vi "TCV1.vi"() -> ()   [LabVIEW 2024]
uses:
  <vilib>/vision/driver/NI_Vision_Acquisition_Software.lvlib
  dependencies_dll_release/TCV_Lib.dll
  <resource>/objmgr/imaqdx.rc
panel:
  in  "CPU:0/Gpu:1":i32=1
  in  "Class name path":path=path "D:/labviewTestTCVdll/TransformCV-LabVIEW/Test/model/candyClasses.txt"
  out "Device Num":u64
  out "success_model_loading":u64
  in  "Model Path":path=path "D:/labviewTestTCVdll/TransformCV-LabVIEW/Test/model/candy11s_1_3_736_1280_gpu.torchscript"
  in  "model_h":i32=736
  in  "iou":dbl=0.65
  in  "conf":dbl=0.6100000000000001 min=0.01 max=1.0 step=0.05
  in  "model_w":i32=1280
  out "height":u32
  out "width":u32
  out "video Mode names":string[](array[string])
  in  "Resolution Selection":u16(ring)=10 items=["640x480 MJPG 30.00fps", "1280x720 MJPG 30.00fps", "1920x1080 MJPG 30.00fps", "1920x1088 MJPG 30.00fps"]
  in  "Camera Selection":string(combo)="cam5"
  in  "confirm camera":bool
  out "Camera Index list":string[](array[string])
  out "Camera":T1(plugin-control)
  in  "stop":bool
  out "return type":i32
  out "no_of_detections":i32
  out "arry_cluster":T2(array[cluster])
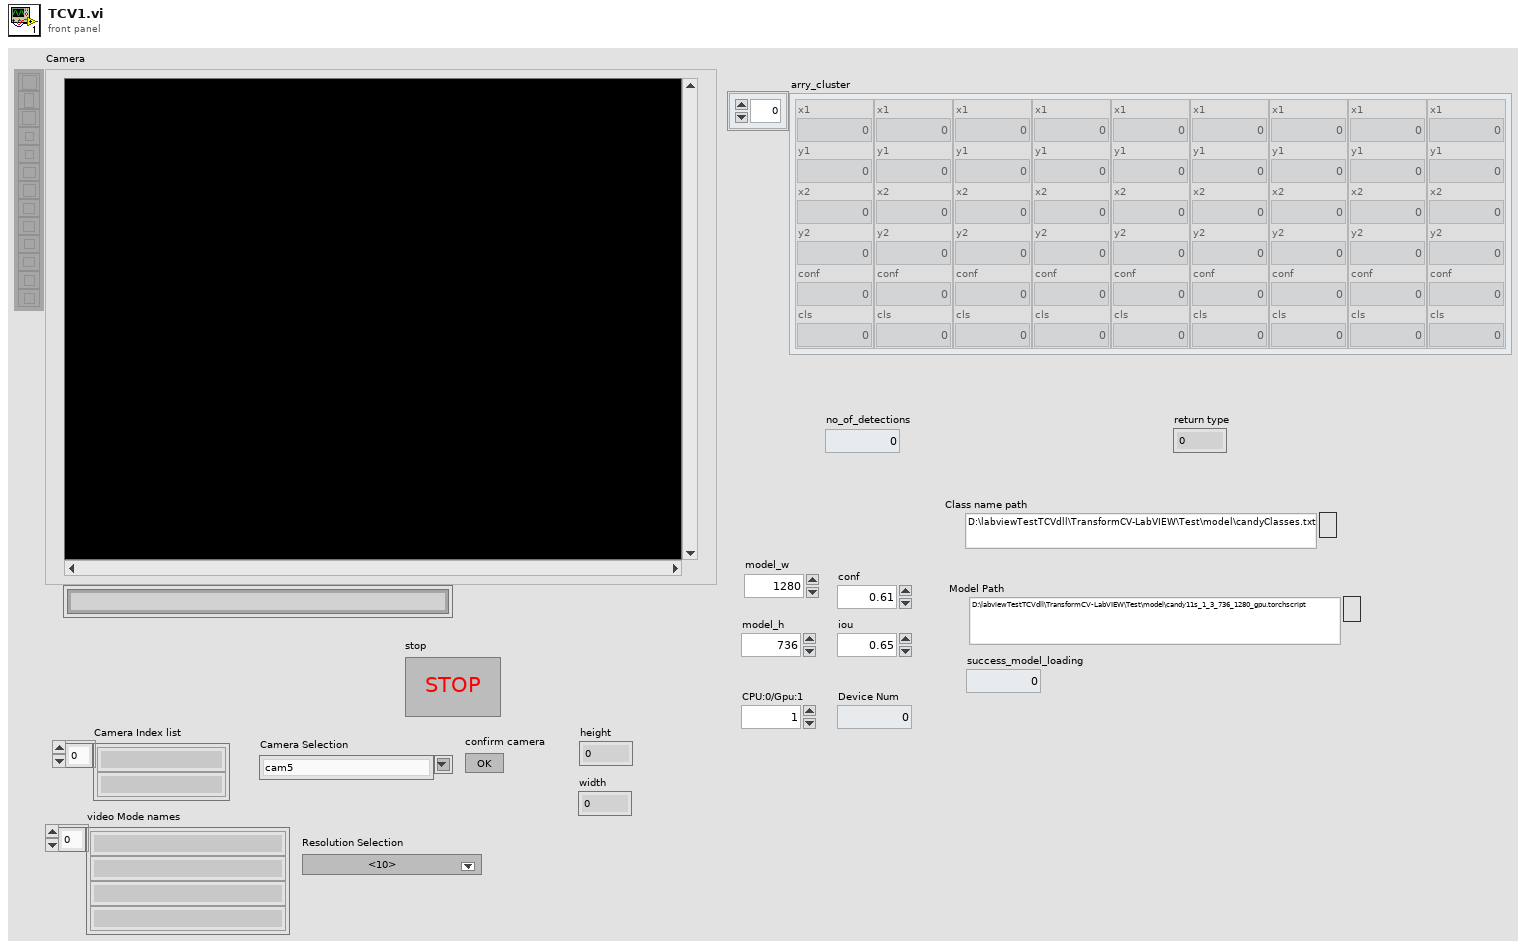
[diagram p1: front panel]
types:
  T1 = typedef "IMAQ Image.ctl" = refnum<image>
  T2 = cluster{"x1":sgl, "y1":sgl, "x2":sgl, "y2":sgl, "conf":sgl, "cls":i32}[]
  T3 = cluster{"Type":u32, "Version":u32, "Flags":u32, "SerialNumberHigh":u32, "SerialNumberLow":u32, "BusType":u32, "InterfaceName":string, "VendorName":string, "ModelName":string, "CameraFileName":string, "CameraAttributeURL":string}[]
  T4 = typedef "IMAQdx.ctl" = refnum<k21>
  T5 = cluster{"Video Mode":u32, "Video Mode Name":string}[]
  T6 = cluster{"x1":sgl, "y1":sgl, "x2":sgl, "y2":sgl, "conf":sgl, "cls":i32}
  T7 = enum32{"Map Pixel Pointer", "Unmap Pixel Pointer", "Get Pixels Infos"}
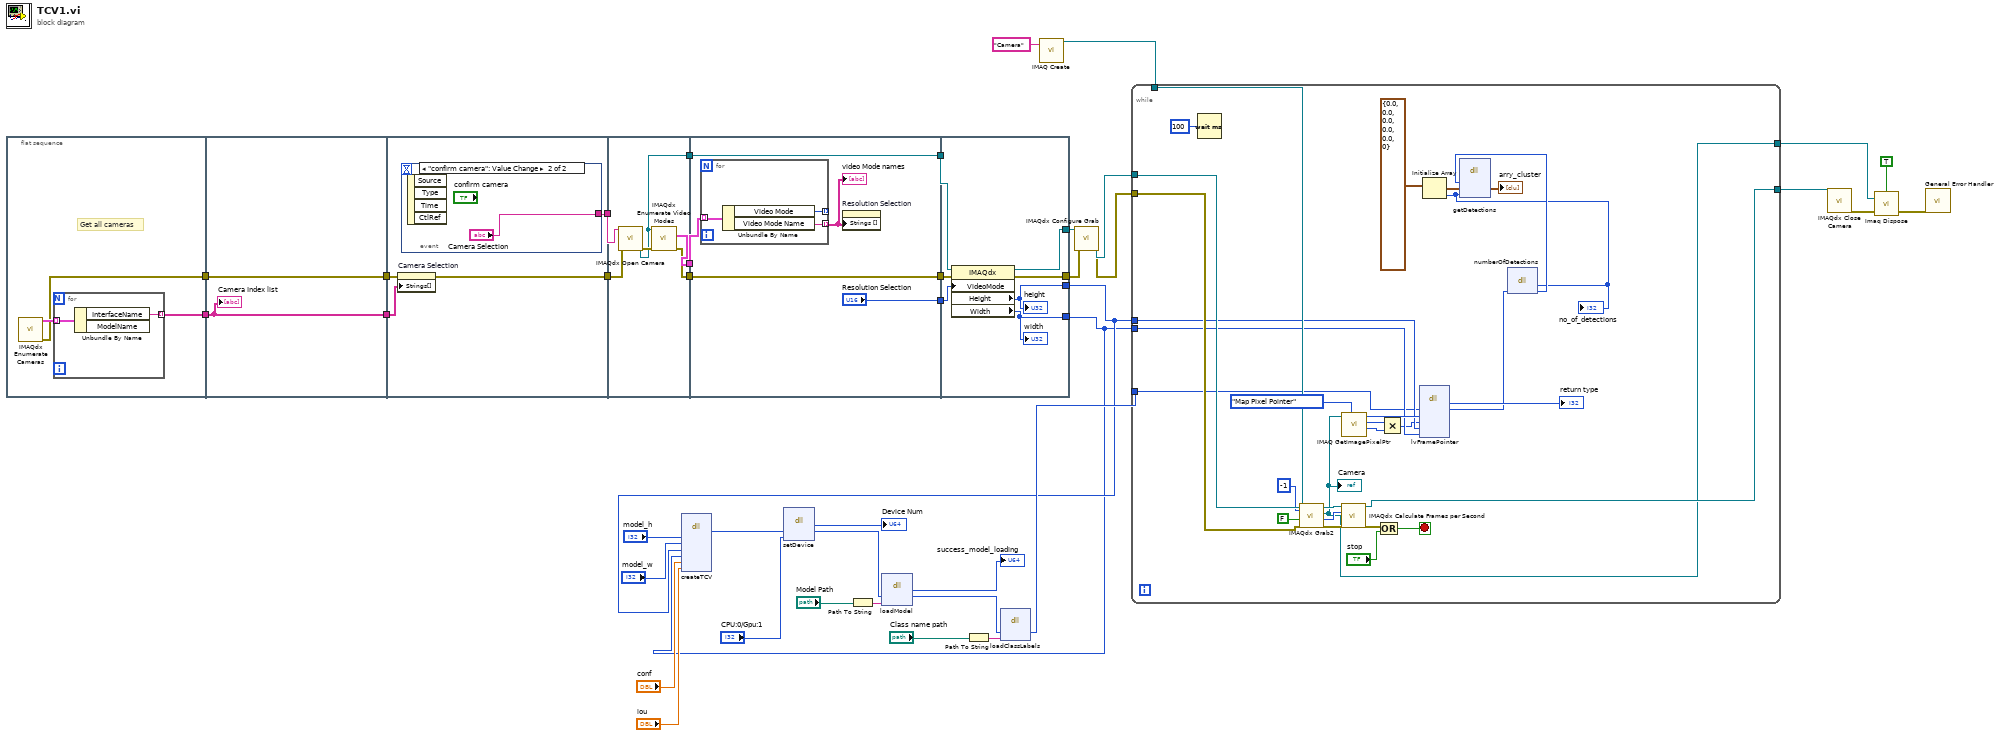
[diagram p0: block diagram]
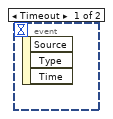
[diagram p2: hidden frame]
diagram:
  n1 = flat-sequence {
    tunnel: [w43] -> w40
    tunnel: [w41] -> w39
    tunnel: w40 -> [w47]
    tunnel: [w47] -> w38
    tunnel: [w46] -> w37
    tunnel: w39 -> [w46]
    tunnel: w38 -> [w51]
    tunnel: w37 -> [w50]
    tunnel: [w48] -> w36
    tunnel: [w49] -> w35
    tunnel: w36 -> [w58]
    tunnel: w35 -> [w57]
    tunnel: [w55] -> w34
    tunnel: [w54] -> w33
    tunnel: [w53] -> w32
    tunnel: w34 -> [w63]
    tunnel: [w61] -> w31
    tunnel: w33 -> [w61]
    tunnel: ["Resolution Selection"] -> w30
    tunnel: [w59] -> w29
    tunnel: w32 -> [w59]
    tunnel: w31 -> [w73]
    tunnel: w30 -> [w72]
    tunnel: w29 -> [w71]
    tunnel: [w70] -> w1
    tunnel: [w69] -> w2
    tunnel: [w68] -> w19
    tunnel: [w67] -> w18
    frame #0 {
      # "Get all cameras"
      n2 = call <vilib>:"IMAQdx Enumerate Cameras.vi"() -> ("error out"=w41:errorcluster, "Camera Information Array"=w42:T3)  [unwired: 10 in]
      n3 = for {
        tunnel: w42 -> [w45] mode=indexing
        tunnel: [w44] -> w43 mode=indexing
        n4 = Unbundle By Name(w45) -> ("InterfaceName"=w44:string)  [unwired: 1 out]
      }
    }
    frame #1 {
      "Camera Index list" <- w47
    }
    frame #2 {
      n5 = property on="Camera Selection" class="CmbBox"(error in=w50, "Strings[]"=w51) -> (error out=w49:errorcluster)  [unwired: 1 in, 1 out]
      n6 = event shown="[1] \"confirm camera\": Value Change" {
        selector: _ -> [_ _]
        dyn-events: _ -> [_ _]
        timeout: _ -> [_ _]
        tunnel: [_ "Camera Selection"] -> w48
        event Timeout {
          n7 = event-data() -> ()  [unwired: 1 in, 3 out]
        }
        event "confirm camera": Value Change {
          n8 = event-data() -> ()  [unwired: 1 in, 4 out]
        }
      }
    }
    frame #3 {
      n9 = call <vilib>:"IMAQdx Open Camera.vi"("error in"=w57, "Session In"=w58) -> ("error out"=w56:errorcluster, "Session Out"=w54:T4)  [unwired: 8 in]
      n10 = call <vilib>:"IMAQdx Enumerate Video Modes.vi"("error in"=w56, "Session In"=w54) -> ("error out"=w53:errorcluster, "Video Modes"=w55:T5)  [unwired: 6 in, 2 out]
    }
    frame #4 {
      n11 = for {
        tunnel: w63 -> [w66] mode=indexing
        tunnel: [w65] -> _ mode=indexing
        tunnel: [w64] -> w62 mode=indexing
        n12 = Unbundle By Name(w66) -> ("Video Mode"=w65:u32, "Video Mode Name"=w64:string)
      }
      "video Mode names" <- w62
      n13 = property on="Resolution Selection" class="Ring (strict)"("Strings []"=w62) -> ()  [unwired: 2 in, 2 out]
    }
    frame #5 {
      n14 = property class="IMAQdx"(reference=w73, error in=w71, "VideoMode"=w72) -> (reference out=w68:T4, error out=w67:errorcluster, "Height"=w69:u32, "Width"=w70:u32)
      "height" <- w69
      "width" <- w70
    }
  }
  n15 = dll-call lib="D:/labviewTestTCVdll/TransformCV-LabVIEW/Test/dependencies_dll_release/TCV_Lib.dll" fn="createTCV"("model_h"="model_h", "model_w"="model_w", "frame_h"=w2, "frame_w"=w1, "conf"="conf", "iou"="iou") -> ("return Obj"=w11:u64)  [unwired: 9 in, 2 out]
  n16 = dll-call lib="D:/labviewTestTCVdll/TransformCV-LabVIEW/Test/dependencies_dll_release/TCV_Lib.dll" fn="setDevice"("ref"=w11, "device"="CPU:0/Gpu:1") -> ("return type"=→"Device Num":u64, "ref"=w8:u64)  [unwired: 4 in, 2 out]
  n17 = Path To String(path="Model Path") -> (string=w12:string)
  n18 = dll-call lib="D:/labviewTestTCVdll/TransformCV-LabVIEW/Test/dependencies_dll_release/TCV_Lib.dll" fn="loadModel"("ref"=w8, "path"=w12) -> ("success"=→"success_model_loading":i32, "ref"=w5:u64)  [unwired: 4 in, 2 out]
  n19 = Path To String(path="Class name path") -> (string=w6:string)
  n20 = dll-call lib="D:/labviewTestTCVdll/TransformCV-LabVIEW/Test/dependencies_dll_release/TCV_Lib.dll" fn="loadClassLabels"("ref"=w5, "class_names"=w6) -> ("ref"=w3:u64)  [unwired: 5 in, 2 out]
  n21 = call "IMAQ Create"("Image Name"="Camera") -> ("New Image"=w25:T1)  [unwired: 4 in, 1 out]
  n22 = call <vilib>:"IMAQdx Configure Grab.vi"("error in"=w18, "Session In"=w19) -> ("error out"=w26:errorcluster, "Session Out"=w27:T4)  [unwired: 8 in]
  n23 = while {
    tunnel: w27 -> [w99]
    tunnel: w26 -> [w97]
    tunnel: w25 -> [w98]
    tunnel: [w91] -> w24
    tunnel: [w84] -> w23
    tunnel: w2 -> [w86]
    tunnel: w1 -> [w85]
    tunnel: w3 -> [w81]
    stop <- w102 stop-if-true
    n24 = Wait (ms)(milliseconds to wait=u32 100) -> ()  [unwired: 1 out]
    n25 = call <vilib>:"IMAQdx Grab2.vi"("Timeout (ms)"=-1, "error in"=w97, "Wait for Next Buffer? (Yes)"=FALSE, "Image In"=w98, "Session In"=w99) -> ("error out"=w92:errorcluster, "Buffer Number Out"=w94:u32, "Image Out"=w84:T1, "Session Out"=w95:T4)  [unwired: 3 in]
    "Camera" <- w84
    n26 = call <vilib>:"IMAQdx Calculate Frames per Second.vi"("Session In"=w95, "Buffer Number"=w94, "error in (no error)"=w92) -> ("Session Out"=w91:T4, "error out"=w89:errorcluster)  [unwired: 6 in, 5 out]
    n27 = call "IMAQ GetImagePixelPtr"("Function"=T7."Map Pixel Pointer", "Image"=w84) -> ("Pixel Size (Bytes)"=w83:i32, "LineWidth(Pixels)"=w88:i32, "Pixel Pointer out"=w87:u64)  [unwired: 4 in, 3 out]
    n28 = Or(x=w89, y="stop") -> (x .or. y?=w102:bool)
    n29 = Multiply(x=w88, y=w83) -> (x*y=w82:i32)
    n30 = dll-call lib="D:/labviewTestTCVdll/TransformCV-LabVIEW/Test/dependencies_dll_release/TCV_Lib.dll" fn="lvFramePointer"("ref"=w81, "ImagePointer"=w87, "Linewidth"=w82, "h"=w86, "w"=w85) -> ("return type"=→"return type":i32, "ref"=w74:u64)  [unwired: 7 in, 2 out]
    n31 = dll-call lib="D:/labviewTestTCVdll/TransformCV-LabVIEW/Test/dependencies_dll_release/TCV_Lib.dll" fn="numberOfDetections"("ref"=w74) -> ("no_of_detections"=w75:i32, "ref"=w76:u64)  [unwired: 3 in, 2 out]
    "no_of_detections" <- w75
    n32 = Initialize Array(T6 {"x1"=0.0, "y1"=0.0, "x2"=0.0, "y2"=0.0, "conf"=0.0, "cls"=0}, w75) -> (w78:T2)
    n33 = dll-call lib="D:/labviewTestTCVdll/TransformCV-LabVIEW/Test/dependencies_dll_release/TCV_Lib.dll" fn="getDetections"("ref"=w76, "arry_cluster"=w78, "numberofdetection"=w75) -> ("arry_cluster"=→"arry_cluster":T2)  [unwired: 6 in, 2 out]
  }
  n34 = call <vilib>:"IMAQdx Close Camera.vi"("Session In"=w24) -> ("error out"=w22:errorcluster)  [unwired: 10 in]
  n35 = call "Imaq Dispose"("All Images? (No)"=TRUE, "Image"=w23, "error in (no error)"=w22) -> ("error out"=w21:errorcluster)  [unwired: 3 in]
  n36 = call <vilib>:"General Error Handler.vi"("error in (no error)"=w21) -> ()  [unwired: 10 in, 5 out]
